vi "MongoDB.EnumerateIEnum.vi"(8 "error in (no error)":errorcluster, 11 ".NET Refnum in":refnum<k24>) -> (0 "error out":errorcluster, 3 "Array":string[](array[string]))   [LabVIEW 2014]
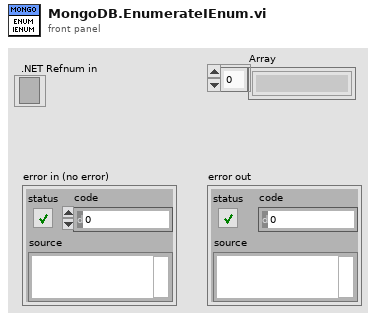
[diagram p1: front panel]
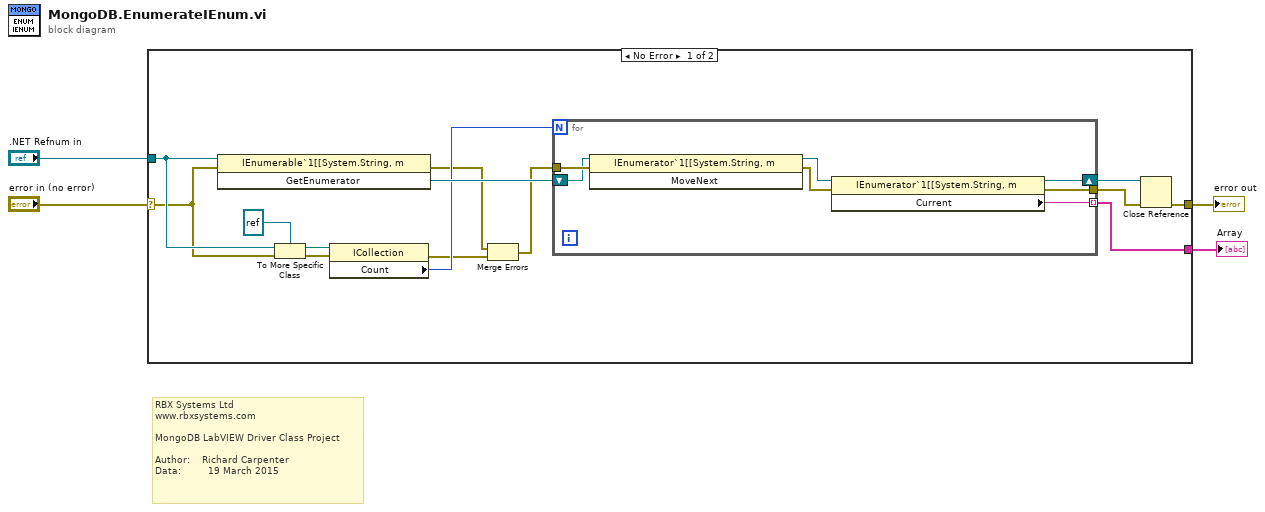
[diagram p0: block diagram]
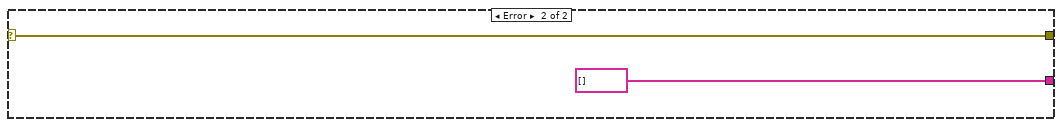
[diagram p2: hidden frame]
diagram:
  # "RBX Systems Ltd\nwww.rbxsystems.com\n\nMongoDB LabVIEW Driver Class Project\n\nAuthor:    Richard Carpenter\nData:         19 March 2015"
  n1 = case shown="No Error" "error in (no error)" {
    selector: "error in (no error)" -> [w5 w27]
    tunnel: [w18 w27] -> w4
    tunnel: [w15 string[] []] -> w3
    tunnel: ".NET Refnum in" -> [w8 _]
    frame No Error {
      n2 = invoke class="IEnumerable`1[[System.String, m" method="GetEnumerator"(reference=w8, error in=w5) -> (error out=w9:errorcluster, "GetEnumerator"=w14:refnum<k24>)  [unwired: 1 in, 1 out]
      n3 = To More Specific Class(target class=refnum<k24> refnum ("ICollection"), reference=w8, error in=w5) -> (specific class reference=w7:refnum<k24>, error out=w12:errorcluster)
      n4 = property class="ICollection"(reference=w7, error in=w12) -> (error out=w10:errorcluster, "Count"=w13:i32)  [unwired: 1 out]
      n5 = Merge Errors(w9, w10) -> (w11:errorcluster)
      n6 = for {
        N: w13 -> [_]
        tunnel: w11 -> [w21]
        shift-right: [w24] -> w16
        shift-left: w14 -> [w19]
        tunnel: [w25] -> w15 mode=indexing
        tunnel: [w23] -> w17
        n7 = invoke class="IEnumerator`1[[System.String, m" method="MoveNext"(reference=w19, error in=w21) -> (reference out=w22:refnum<k24>, error out=w20:errorcluster)  [unwired: 1 in, 1 out]
        n8 = property class="IEnumerator`1[[System.String, m"(reference=w22, error in=w20) -> (reference out=w24:refnum<k24>, error out=w23:errorcluster, "Current"=w25:string)
      }
      n9 = Close Reference(reference=w16, error in (no error)=w17) -> (error out=w18:errorcluster)
    }
    frame Error {
    }
  }
  "error out" <- w4
  "Array" <- w3
